vi "EG_G5210 Read Param.vi"(8 "error in (no error)":errorcluster, 9 "Énum":T3, 10 "LockInPar In":T1={"Sensitivity"=13, "Vernier Mode"=FALSE, "Vernier Value"=0, "Main Filter"=3, "Filter Freq (Hz)"=0.0, "Filter Mode"=1, " Line Notch"=3, "Reference"=1, "Reference Mode"=0, "Ref Phase (°)"=0.0, "Ref Freq (Hz)"=0.0, "Output Filter"=0, "Time Constant"=13, "Dynamic Res."=1, "X Offset"=FALSE, "X Offset Val %"=0.0, "Y Offset"=FALSE, "Y Offset Val %"=0.0, "Expand"=FALSE, "Osc Amp. (mV rms)"=0, "Int Osc (Hz)"=0.0, "Trigger Mode"=0, "Input Mode"=0, "Ovld Source"=0} caption="Lock-In Parameters In" {"Ovld Source" items=["None", "Y Channel", "X Channel", "PSD", "Input", "Ref Unlck"]; "Input Mode" items=["Current 10E8 A/V", "Current 10E6 A/V", "Voltage"]; "Trigger Mode" items=["Reference", "External", "Asynchronous", "Ratio", "8F"]; "Reference Mode" items=["F", "2F"]; "Reference" items=["External", "Internal"]; "Filter Mode" items=["Manual", "Automatic"]; "Line Notch" items=["Off", "120 Hz", "60 Hz", "Both"]; "Main Filter" items=["No Filter", "Notch", "Low Pass", "Band Pass"]; "Output Filter" items=["6dB", "12dB"]; "Time Constant" items=["1 ms", "3 ms", "10 ms", "30 ms", "100 ms", "300 ms", "1 s", "3 s", "10 s", "30 s", "100 s", "300 s", "1000 s", "3000 s"]; "Sensitivity" items=["100 nV", "300 nV", "1 µV", "3 µV", "10 µV", "30 µV", "100µV", "300 µV", "1 mV", "3 mV", "10 mV", "30 mV", "100 mV", "300 mV", "1 V", "3 V"]; "Dynamic Res." items=["Hi Stab", "Normal", "Hi Res"]}, 11 "Ressource VISA":refnum<visa-resource-name>="GPIB0::8::INSTR") -> (0 "error out":errorcluster, 1 "LockInPar":T1={"Sensitivity"=1, "Vernier Mode"=FALSE, "Vernier Value"=0, "Main Filter"=0, "Filter Freq (Hz)"=0.0, "Filter Mode"=0, " Line Notch"=0, "Reference"=0, "Reference Mode"=0, "Ref Phase (°)"=0.0, "Ref Freq (Hz)"=0.0, "Output Filter"=0, "Time Constant"=1, "Dynamic Res."=0, "X Offset"=FALSE, "X Offset Val %"=0.0, "Y Offset"=FALSE, "Y Offset Val %"=0.0, "Expand"=FALSE, "Osc Amp. (mV rms)"=0, "Int Osc (Hz)"=0.0, "Trigger Mode"=0, "Input Mode"=0, "Ovld Source"=0} caption="Lock-In Parameters Out" {"Ovld Source" items=["None", "Y Channel", "X Channel", "PSD", "Input", "Ref Unlck"]; "Input Mode" items=["Current 10E8 A/V", "Current 10E6 A/V", "Voltage"]; "Trigger Mode" items=["Reference", "External", "Asynchronous", "Ratio", "8F"]; "Reference Mode" items=["F", "2F"]; "Reference" items=["External", "Internal"]; "Filter Mode" items=["Manual", "Automatic"]; "Line Notch" items=["Off", "120 Hz", "60 Hz", "Both"]; "Main Filter" items=["No Filter", "Notch", "Low Pass", "Band Pass"]; "Output Filter" items=["6dB", "12dB"]; "Time Constant" items=["1 ms", "3 ms", "10 ms", "30 ms", "100 ms", "300 ms", "1 s", "3 s", "10 s", "30 s", "100 s", "300 s", "1000 s", "3000 s"]; "Sensitivity" items=["100 nV", "300 nV", "1 µV", "3 µV", "10 µV", "30 µV", "100µV", "300 µV", "1 mV", "3 mV", "10 mV", "30 mV", "100 mV", "300 mV", "1 V", "3 V"]; "Dynamic Res." items=["Hi Stab", "Normal", "Hi Res"]}, 2 "Params":string, 3 "Ressource VISA Out":refnum<visa-resource-name>="GPIB0::8::INSTR")   [LabVIEW 2019]
uses:
  <userlib>/EG_G 5210 LIA/LockInPar.ctl
  <userlib>/EG_G 5210 LIA/TrigMode.ctl
  <userlib>/EG_G 5210 LIA/ReadFunctions.ctl
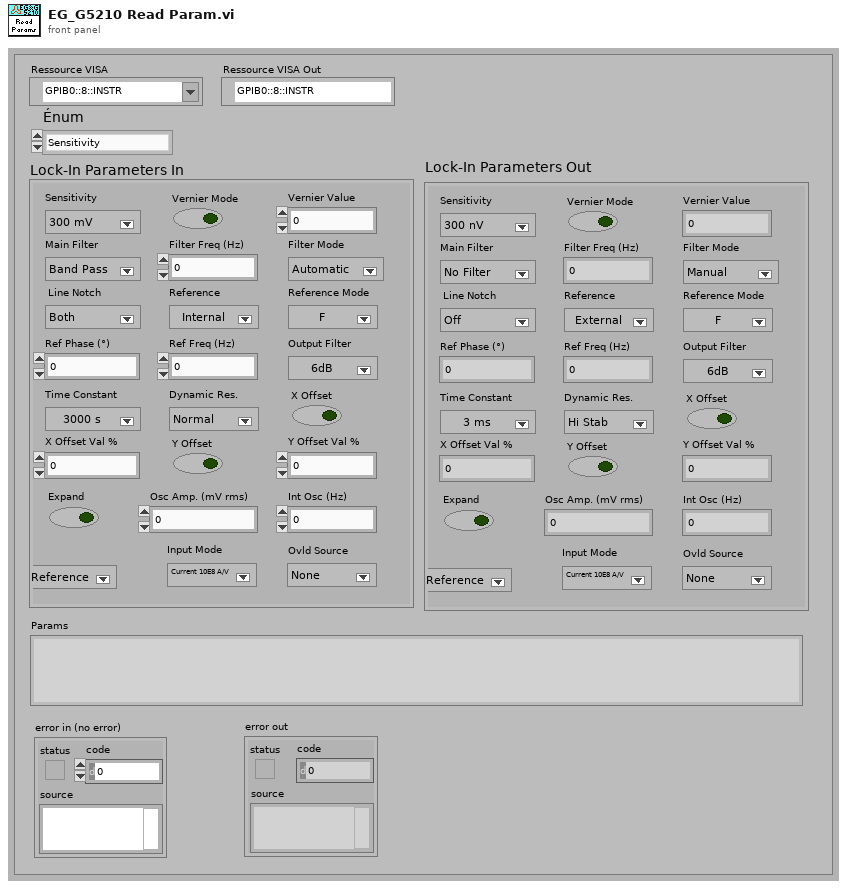
[diagram p1: front panel]
types:
  T1 = typedef "LockInPar.ctl" = cluster{"Sensitivity":u16, "Vernier Mode":bool, "Vernier Value":i32, "Main Filter":u16, "Filter Freq (Hz)":dbl, "Filter Mode":u16, " Line Notch":u16, "Reference":u16, "Reference Mode":u16, "Ref Phase (°)":dbl, "Ref Freq (Hz)":dbl, "Output Filter":u16, "Time Constant":u16, "Dynamic Res.":u16, "X Offset":bool, "X Offset Val %":dbl, "Y Offset":bool, "Y Offset Val %":dbl, "Expand":bool, "Osc Amp. (mV rms)":i32, "Int Osc (Hz)":dbl, "Trigger Mode":T2, "Input Mode":u16, "Ovld Source":u16}
  T2 = typedef "TrigMode.ctl" = u16
  T3 = typedef "ReadFunctions.ctl" = enum16{"Sensitivity", "Vernier Mode", "Main Filter", "Filter Mode", "Line Filter", "Ref Source", "Ref Mode", "Ref Phase", "Ref Frequency", "Output Filter", "Time Constant", "Dyn Reserve", "X Offset", "Y Offset", "Expand Mode", "Int Oscillator", "Oscillator Freq", "All params", "Overload Byte", "Trigger Mode", "Error"}
  T4 = enum16{"0.5 Hz to 12 Hz", "10 Hz to 120 Hz", "100 Hz to 1200 Hz", "1 kHz to 12 kHz", "10 kHz to 120 kHz"}
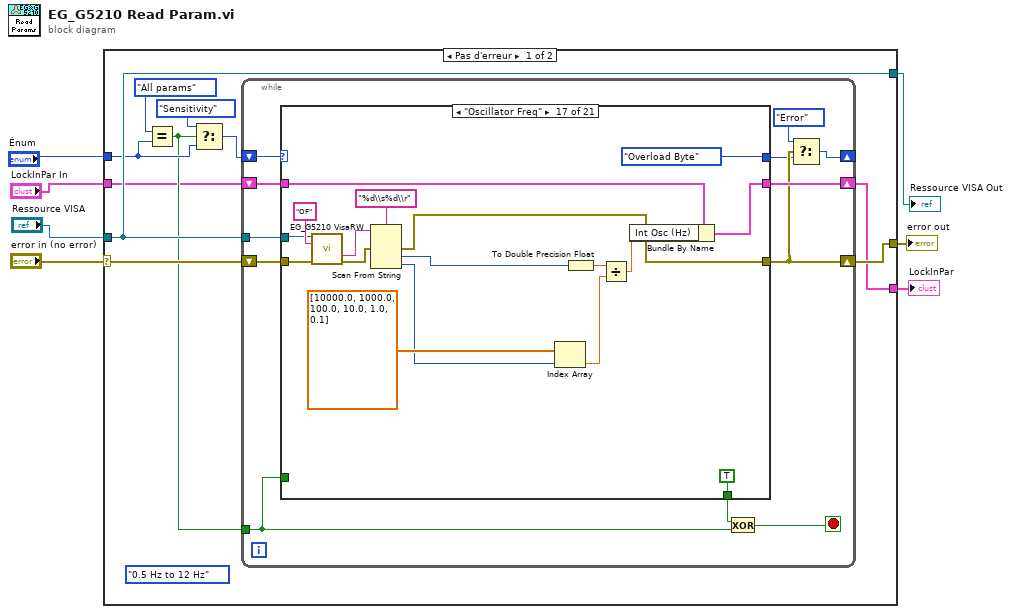
[diagram p0: block diagram]
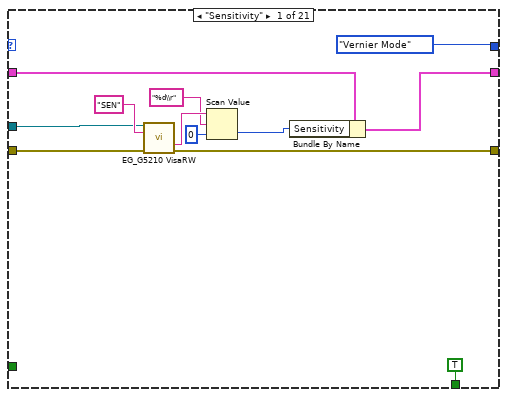
[diagram p2: hidden frame]
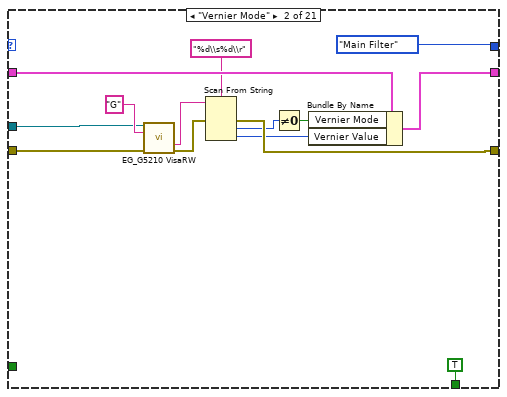
[diagram p3: hidden frame]
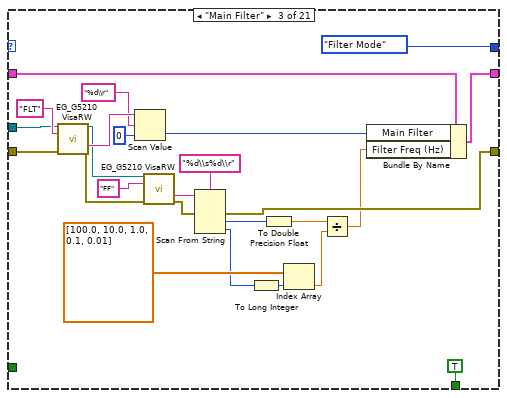
[diagram p4: hidden frame]
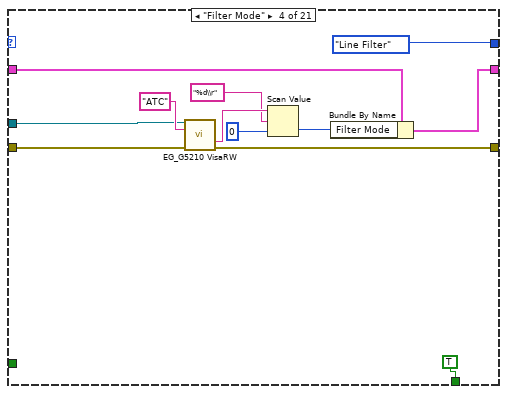
[diagram p5: hidden frame]
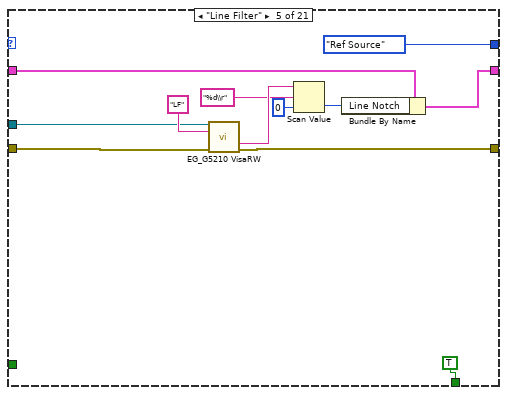
[diagram p6: hidden frame]
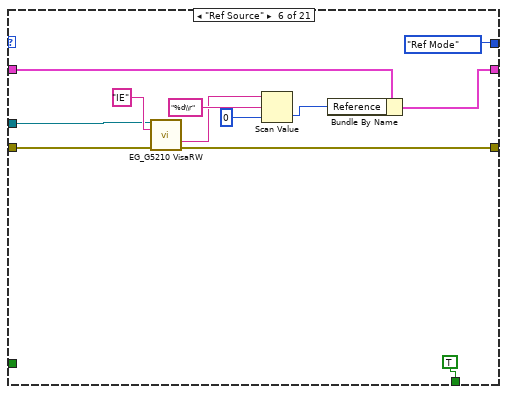
[diagram p7: hidden frame]
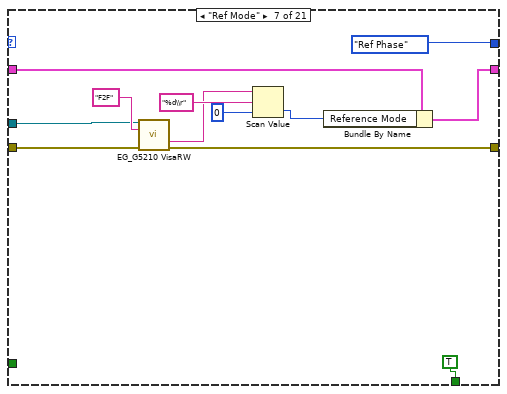
[diagram p8: hidden frame]
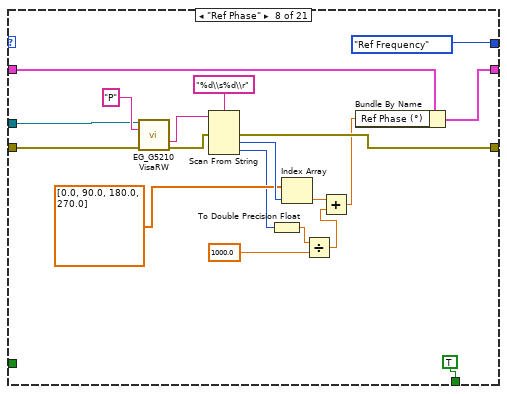
[diagram p9: hidden frame]
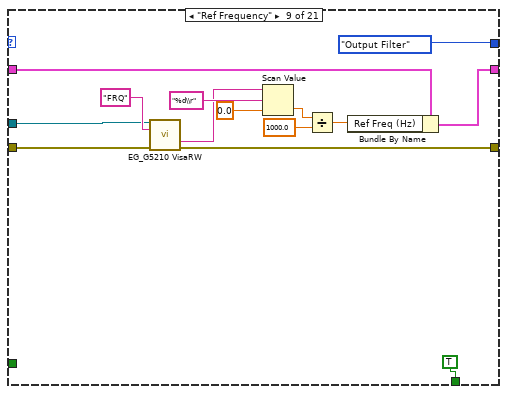
[diagram p10: hidden frame]
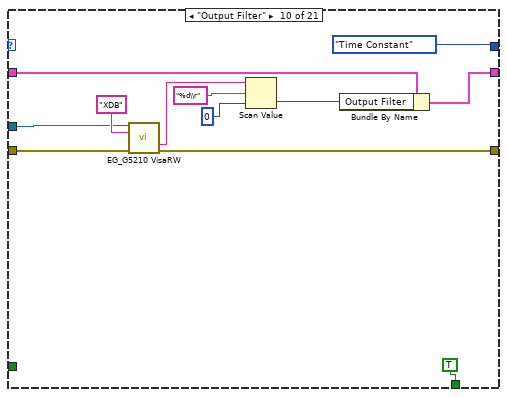
[diagram p11: hidden frame]
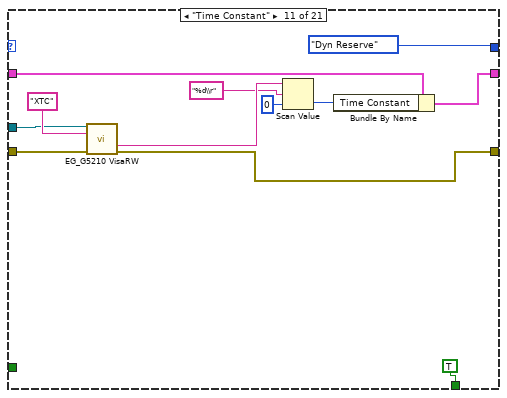
[diagram p12: hidden frame]
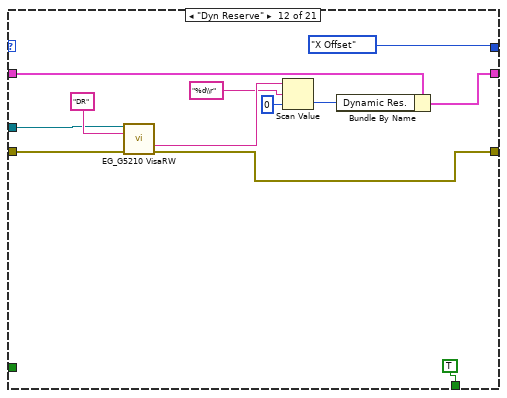
[diagram p13: hidden frame]
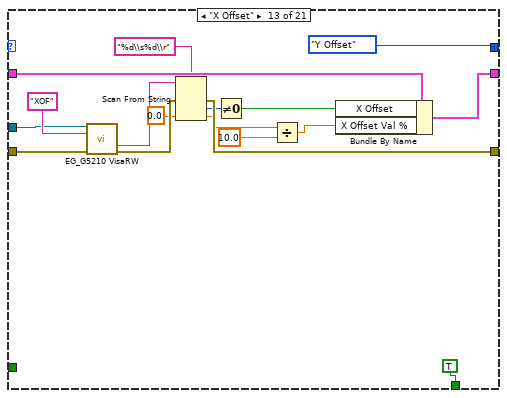
[diagram p14: hidden frame]
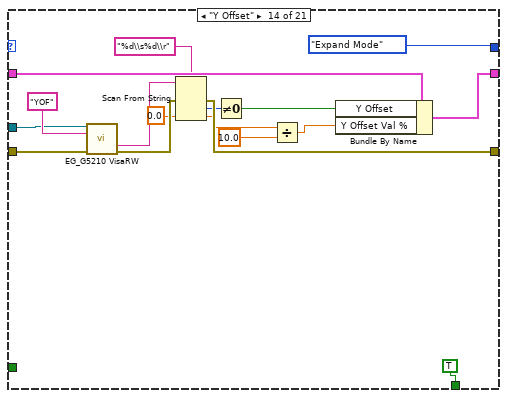
[diagram p15: hidden frame]
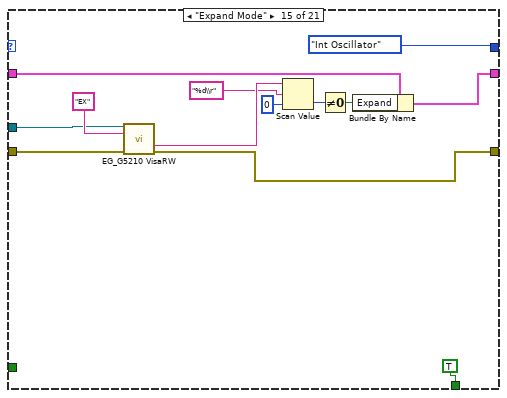
[diagram p16: hidden frame]
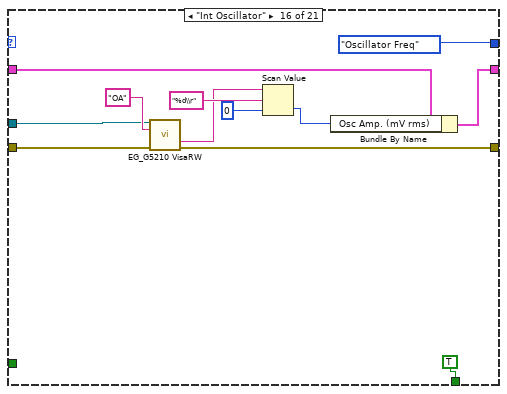
[diagram p17: hidden frame]
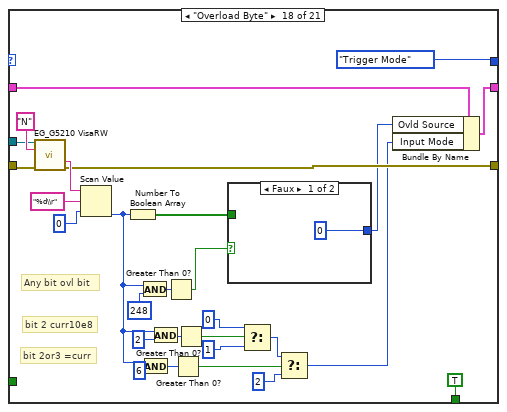
[diagram p18: hidden frame]
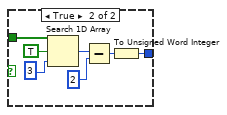
[diagram p19: hidden frame]
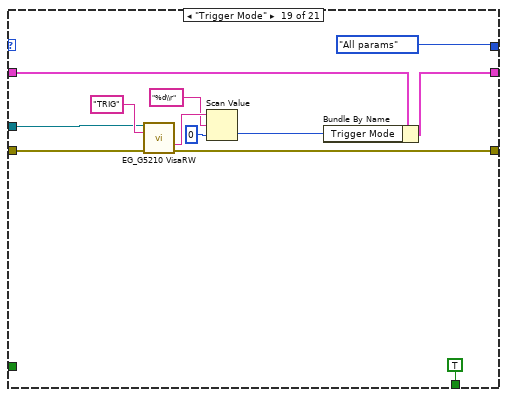
[diagram p20: hidden frame]
diagram:
  n1 = case shown="Pas d'erreur" "error in (no error)" {
    selector: "error in (no error)" -> [w16 w334]
    tunnel: [w17 w334] -> w6
    tunnel: [w15 w333] -> w5
    tunnel: "Ressource VISA" -> [w15 w333]
    tunnel: [w14 _] -> w3
    tunnel: "Énum" -> [w11 _]
    tunnel: "LockInPar In" -> [w8 _]
    frame No Error {
      (unwired) T4."0.5 Hz to 12 Hz"
      n2 = Equal?(x=ReadFunctions."All params" ("Énum"), y=w11) -> (x = y?=w9:bool)
      n3 = Select(t=ReadFunctions."Sensitivity" ("Énum"), s=w9, f=w11) -> (s? t:f=w10:T3)
      n4 = while {
        shift-right: [w19] -> _
        shift-left: w10 -> [w29]
        shift-right: [w21] -> w17
        shift-left: w16 -> [w28]
        tunnel: w15 -> [w27]
        shift-right: [w26] -> w14
        shift-left: w8 -> [w25]
        tunnel: w9 -> [w22]
        stop <- w23 stop-if-true
        n5 = case shown="\"Oscillator Freq\"" w29 {
          selector: w29 -> [_ _ _ _ _ _ _ _ _ _ _ _ _ _ _ _ _ _ _ _ w332]
          tunnel: w28 -> [w38 w54 w79 w91 w100 w115 w127 w146 w160 w172 w182 w194 w212 w229 w241 w255 w272 w298 w318 w326 w331]
          tunnel: [w36 w45 w59 w90 w94 w114 w126 w137 w159 w162 w174 w186 w205 w222 w233 w254 w258 w296 w316 w325 w331] -> w21
          tunnel: w27 -> [w37 w53 w78 w89 w101 w113 w125 w145 w158 w171 w181 w193 w211 w228 w240 w253 w271 w297 w317 _ _]
          tunnel: [ReadFunctions."Vernier Mode" ReadFunctions."Main Filter" ReadFunctions."Filter Mode" ReadFunctions."Line Filter" ReadFunctions."Ref Source" ReadFunctions."Ref Mode" ReadFunctions."Ref Phase" ReadFunctions."Ref Frequency" ReadFunctions."Output Filter" ReadFunctions."Time Constant" ReadFunctions."Dyn Reserve" ReadFunctions."X Offset" ReadFunctions."Y Offset" ReadFunctions."Expand Mode" ReadFunctions."Int Oscillator" ReadFunctions."Oscillator Freq" ReadFunctions."Overload Byte" ReadFunctions."Trigger Mode" ReadFunctions."All params" ReadFunctions."Vernier Mode" w332] -> w20
          tunnel: [TRUE TRUE TRUE TRUE TRUE TRUE TRUE TRUE TRUE TRUE TRUE TRUE TRUE TRUE TRUE TRUE TRUE TRUE TRUE FALSE w329] -> w24
          tunnel: w25 -> [w31 w49 w73 w83 w96 w110 w122 w142 w154 w166 w177 w189 w208 w225 w236 w249 w269 w292 w312 w322 w328]
          tunnel: [w32 w50 w57 w84 w97 w109 w121 w141 w155 w165 w176 w188 w207 w224 w235 w250 w268 w293 w313 w322 w328] -> w26
          tunnel: w22 -> [_ _ _ _ _ _ _ _ _ _ _ _ _ _ _ _ _ _ _ _ w330]
          frame "Sensitivity" {
            n6 = call <userlib>:"EG_G5210 VisaRW.vi"("VISA Rsrc"=w37, "ChaineCom"="SEN", "error in (no error)"=w38) -> ("ChaineRep"=w40:string, "error out"=w36:errorcluster)  [unwired: 9 in, 2 out]
            n7 = Scan Value(string=w40, format string="%d\\r" ("chaîne de format"), default (0 dbl)=u16 0 ("valeur par défaut (0 I32)")) -> (value=w33:u16)  [unwired: 1 out]
            n8 = Bundle By Name(cluster=w31, "Sensitivity"=w33) -> (w32:T1)
          }
          frame "Vernier Mode" {
            n9 = call <userlib>:"EG_G5210 VisaRW.vi"("VISA Rsrc"=w53, "ChaineCom"="G", "error in (no error)"=w54) -> ("ChaineRep"=w47:string, "error out"=w46:errorcluster)  [unwired: 9 in, 2 out]
            n10 = Scan From String(format string="%d\\s%d\\r" ("chaîne de format"), input string=w47, error in=w46) -> (error out=w45:errorcluster, output 1=w44:i32, output 2=w42:i32)  [unwired: 3 in, 2 out]
            n11 = Not Equal To 0?(x=w44) -> (x != 0?=w43:bool)
            n12 = Bundle By Name(cluster=w49, "Vernier Mode"=w43, "Vernier Value"=w42) -> (w50:T1)
          }
          frame "Main Filter" {
            n13 = call <userlib>:"EG_G5210 VisaRW.vi"("VISA Rsrc"=w78, "ChaineCom"="FLT", "error in (no error)"=w79) -> ("VISA Rsrc Out"=w71:refnum<visa-resource-name>, "ChaineRep"=w77:string, "error out"=w70:errorcluster)  [unwired: 9 in, 1 out]
            n14 = Scan Value(string=w77, format string="%d\\r" ("chaîne de format"), default (0 dbl)=u16 0 ("valeur par défaut (0 I32)")) -> (value=w72:u16)  [unwired: 1 out]
            n15 = call <userlib>:"EG_G5210 VisaRW.vi"("VISA Rsrc"=w71, "ChaineCom"="FF", "error in (no error)"=w70) -> ("ChaineRep"=w68:string, "error out"=w60:errorcluster)  [unwired: 9 in, 2 out]
            n16 = Scan From String(format string="%d\\s%d\\r" ("chaîne de format"), input string=w68, error in=w60) -> (error out=w59:errorcluster, output 1=w62:i32, output 2=w61:i32)  [unwired: 3 in, 2 out]
            n17 = To Long Integer(number=w61) -> (32bit integer=w65:i32)
            n18 = To Double Precision Float(number=w62) -> (double precision float=w63:dbl)
            n19 = Index Array(array=dbl[] [100.0, 10.0, 1.0, 0.1, 0.01], index=w65) -> (element=w66:dbl)
            n20 = Divide(x=w63, y=w66) -> (x/y=w56:dbl)
            n21 = Bundle By Name(cluster=w73, "Main Filter"=w72, "Filter Freq (Hz)"=w56) -> (w57:T1)
          }
          frame "Filter Mode" {
            n22 = call <userlib>:"EG_G5210 VisaRW.vi"("VISA Rsrc"=w89, "ChaineCom"="ATC", "error in (no error)"=w91) -> ("ChaineRep"=w88:string, "error out"=w90:errorcluster)  [unwired: 9 in, 2 out]
            n23 = Scan Value(string=w88, format string="%d\\r" ("chaîne de format"), default (0 dbl)=u16 0 ("valeur par défaut (0 I32)")) -> (value=w82:u16)  [unwired: 1 out]
            n24 = Bundle By Name(cluster=w83, "Filter Mode"=w82) -> (w84:T1)
          }
          frame "Line Filter" {
            n25 = call <userlib>:"EG_G5210 VisaRW.vi"("VISA Rsrc"=w101, "ChaineCom"="LF", "error in (no error)"=w100) -> ("ChaineRep"=w103:string, "error out"=w94:errorcluster)  [unwired: 9 in, 2 out]
            n26 = Scan Value(string=w103, format string="%d\\r" ("chaîne de format"), default (0 dbl)=u16 0 ("valeur par défaut (0 I32)")) -> (value=w95:u16)  [unwired: 1 out]
            n27 = Bundle By Name(cluster=w96, "Line Notch"=w95) -> (w97:T1)
          }
          frame "Ref Source" {
            n28 = call <userlib>:"EG_G5210 VisaRW.vi"("VISA Rsrc"=w113, "ChaineCom"="IE", "error in (no error)"=w115) -> ("ChaineRep"=w106:string, "error out"=w114:errorcluster)  [unwired: 9 in, 2 out]
            n29 = Scan Value(string=w106, format string="%d\\r" ("chaîne de format"), default (0 dbl)=u16 0 ("valeur par défaut (0 I32)")) -> (value=w105:u16)  [unwired: 1 out]
            n30 = Bundle By Name(cluster=w110, "Reference"=w105) -> (w109:T1)
          }
          frame "Ref Mode" {
            n31 = call <userlib>:"EG_G5210 VisaRW.vi"("VISA Rsrc"=w125, "ChaineCom"="F2F", "error in (no error)"=w127) -> ("ChaineRep"=w118:string, "error out"=w126:errorcluster)  [unwired: 9 in, 2 out]
            n32 = Scan Value(string=w118, format string="%d\\r" ("chaîne de format"), default (0 dbl)=u16 0 ("valeur par défaut (0 I32)")) -> (value=w117:u16)  [unwired: 1 out]
            n33 = Bundle By Name(cluster=w122, "Reference Mode"=w117) -> (w121:T1)
          }
          frame "Ref Phase" {
            n34 = call <userlib>:"EG_G5210 VisaRW.vi"("VISA Rsrc"=w145, "ChaineCom"="P", "error in (no error)"=w146) -> ("ChaineRep"=w139:string, "error out"=w138:errorcluster)  [unwired: 9 in, 2 out]
            n35 = Scan From String(format string="%d\\s%d\\r" ("chaîne de format"), input string=w139, error in=w138) -> (error out=w137:errorcluster, output 1=w136:i32, output 2=w131:i32)  [unwired: 3 in, 2 out]
            n36 = To Double Precision Float(number=w131) -> (double precision float=w132:dbl)
            n37 = Index Array(array=dbl[] [0.0, 90.0, 180.0, 270.0], index=w136) -> (element=w134:dbl)
            n38 = Divide(x=w132, y=1000.0) -> (x/y=w130:dbl)
            n39 = Add(x=w134, y=w130) -> (x+y=w129:dbl)
            n40 = Bundle By Name(cluster=w142, "Ref Phase (°)"=w129) -> (w141:T1)
          }
          frame "Ref Frequency" {
            n41 = call <userlib>:"EG_G5210 VisaRW.vi"("VISA Rsrc"=w158, "ChaineCom"="FRQ", "error in (no error)"=w160) -> ("ChaineRep"=w151:string, "error out"=w159:errorcluster)  [unwired: 9 in, 2 out]
            n42 = Scan Value(string=w151, format string="%d\\r" ("chaîne de format"), default (0 dbl)=0.0 ("valeur par défaut (0 I32)")) -> (value=w150:dbl)  [unwired: 1 out]
            n43 = Divide(x=w150, y=1000.0) -> (x/y=w149:dbl)
            n44 = Bundle By Name(cluster=w154, "Ref Freq (Hz)"=w149) -> (w155:T1)
          }
          frame "Output Filter" {
            n45 = call <userlib>:"EG_G5210 VisaRW.vi"("VISA Rsrc"=w171, "ChaineCom"="XDB", "error in (no error)"=w172) -> ("ChaineRep"=w170:string, "error out"=w162:errorcluster)  [unwired: 9 in, 2 out]
            n46 = Scan Value(string=w170, format string="%d\\r" ("chaîne de format"), default (0 dbl)=u16 0 ("valeur par défaut (0 I32)")) -> (value=w164:u16)  [unwired: 1 out]
            n47 = Bundle By Name(cluster=w166, "Output Filter"=w164) -> (w165:T1)
          }
          frame "Time Constant" {
            n48 = call <userlib>:"EG_G5210 VisaRW.vi"("VISA Rsrc"=w181, "ChaineCom"="XTC", "error in (no error)"=w182) -> ("ChaineRep"=w184:string, "error out"=w174:errorcluster)  [unwired: 9 in, 2 out]
            n49 = Scan Value(string=w184, format string="%d\\r" ("chaîne de format"), default (0 dbl)=u16 0 ("valeur par défaut (0 I32)")) -> (value=w178:u16)  [unwired: 1 out]
            n50 = Bundle By Name(cluster=w177, "Time Constant"=w178) -> (w176:T1)
          }
          frame "Dyn Reserve" {
            n51 = call <userlib>:"EG_G5210 VisaRW.vi"("VISA Rsrc"=w193, "ChaineCom"="DR", "error in (no error)"=w194) -> ("ChaineRep"=w196:string, "error out"=w186:errorcluster)  [unwired: 9 in, 2 out]
            n52 = Scan Value(string=w196, format string="%d\\r" ("chaîne de format"), default (0 dbl)=u16 0 ("valeur par défaut (0 I32)")) -> (value=w190:u16)  [unwired: 1 out]
            n53 = Bundle By Name(cluster=w189, "Dynamic Res."=w190) -> (w188:T1)
          }
          frame "X Offset" {
            n54 = call <userlib>:"EG_G5210 VisaRW.vi"("VISA Rsrc"=w211, "ChaineCom"="XOF", "error in (no error)"=w212) -> ("ChaineRep"=w213:string, "error out"=w206:errorcluster)  [unwired: 9 in, 2 out]
            n55 = Scan From String(format string="%d\\s%d\\r" ("chaîne de format"), input string=w213, error in=w206, default 2=0.0 ("valeur par défaut (0 I32)")) -> (error out=w205:errorcluster, output 1=w204:i32, output 2=w200:dbl)  [unwired: 2 in, 2 out]
            n56 = Not Equal To 0?(x=w204) -> (x != 0?=w202:bool)
            n57 = Divide(x=w200, y=10.0) -> (x/y=w198:dbl)
            n58 = Bundle By Name(cluster=w208, "X Offset"=w202, "X Offset Val %"=w198) -> (w207:T1)
          }
          frame "Y Offset" {
            n59 = call <userlib>:"EG_G5210 VisaRW.vi"("VISA Rsrc"=w228, "ChaineCom"="YOF", "error in (no error)"=w229) -> ("ChaineRep"=w230:string, "error out"=w223:errorcluster)  [unwired: 9 in, 2 out]
            n60 = Scan From String(format string="%d\\s%d\\r" ("chaîne de format"), input string=w230, error in=w223, default 2=0.0 ("valeur par défaut (0 I32)")) -> (error out=w222:errorcluster, output 1=w221:i32, output 2=w217:dbl)  [unwired: 2 in, 2 out]
            n61 = Not Equal To 0?(x=w221) -> (x != 0?=w219:bool)
            n62 = Divide(x=w217, y=10.0) -> (x/y=w215:dbl)
            n63 = Bundle By Name(cluster=w225, "Y Offset"=w219, "Y Offset Val %"=w215) -> (w224:T1)
          }
          frame "Expand Mode" {
            n64 = call <userlib>:"EG_G5210 VisaRW.vi"("VISA Rsrc"=w240, "ChaineCom"="EX", "error in (no error)"=w241) -> ("ChaineRep"=w243:string, "error out"=w233:errorcluster)  [unwired: 9 in, 2 out]
            n65 = Scan Value(string=w243, format string="%d\\r" ("chaîne de format"), default (0 dbl)=u16 0 ("valeur par défaut (0 I32)")) -> (value=w237:u16)  [unwired: 1 out]
            n66 = Not Equal To 0?(x=w237) -> (x != 0?=w232:bool)
            n67 = Bundle By Name(cluster=w236, "Expand"=w232) -> (w235:T1)
          }
          frame "Int Oscillator" {
            n68 = call <userlib>:"EG_G5210 VisaRW.vi"("VISA Rsrc"=w253, "ChaineCom"="OA", "error in (no error)"=w255) -> ("ChaineRep"=w246:string, "error out"=w254:errorcluster)  [unwired: 9 in, 2 out]
            n69 = Scan Value(string=w246, format string="%d\\r" ("chaîne de format"), default (0 dbl)=0 ("valeur par défaut (0 I32)")) -> (value=w245:i32)  [unwired: 1 out]
            n70 = Bundle By Name(cluster=w249, "Osc Amp. (mV rms)"=w245) -> (w250:T1)
          }
          frame "Oscillator Freq" {
            n71 = call <userlib>:"EG_G5210 VisaRW.vi"("VISA Rsrc"=w271, "ChaineCom"="OF", "error in (no error)"=w272) -> ("ChaineRep"=w266:string, "error out"=w265:errorcluster)  [unwired: 9 in, 2 out]
            n72 = Scan From String(format string="%d\\s%d\\r" ("chaîne de format"), input string=w266, error in=w265) -> (error out=w258:errorcluster, output 1=w257:i32, output 2=w259:i32)  [unwired: 3 in, 2 out]
            n73 = Index Array(array=dbl[] [10000.0, 1000.0, 100.0, 10.0, 1.0, 0.1], index=w259) -> (element=w262:dbl)
            n74 = To Double Precision Float(number=w257) -> (double precision float=w264:dbl)
            n75 = Divide(x=w264, y=w262) -> (x/y=w261:dbl)
            n76 = Bundle By Name(cluster=w269, "Int Osc (Hz)"=w261) -> (w268:T1)
          }
          frame "Overload Byte" {
            # "Any bit ovl bit"
            # "bit 2or3 =curr"
            # "bit 2 curr10e8"
            n77 = call <userlib>:"EG_G5210 VisaRW.vi"("VISA Rsrc"=w297, "ChaineCom"="N", "error in (no error)"=w298) -> ("ChaineRep"=w300:string, "error out"=w296:errorcluster)  [unwired: 9 in, 2 out]
            n78 = Scan Value(string=w300, format string="%d\\r" ("chaîne de format"), default (0 dbl)=u16 0 ("valeur par défaut (0 I32)")) -> (value=w277:u16)  [unwired: 1 out]
            n79 = Number To Boolean Array(number=w277) -> (Boolean array=w276:bool[])
            n80 = And(x=w277, y=u16 248) -> (x .and. y?=w279:u16)
            n81 = And(x=w277, y=u16 6) -> (x .and. y?=w287:u16)
            n82 = And(x=w277, y=u16 2) -> (x .and. y?=w286:u16)
            n83 = Greater Than 0?(x=w279) -> (x > 0?=w275:bool)
            n84 = Greater Than 0?(x=w287) -> (x > 0?=w289:bool)
            n85 = Greater Than 0?(x=w286) -> (x > 0?=w284:bool)
            n86 = case shown="Faux" w275 {
              tunnel: w276 -> [_ w308]
              tunnel: [u16 0 w306] -> w274
              frame False {
              }
              frame True {
                n87 = Search 1D Array(1D array=w308, element=TRUE ("élément"), start index (0)=3 ("indice de départ (0)")) -> (index of element=w305:i32)
                n88 = Subtract(x=w305, y=2) -> (x-y=w304:i32)
                n89 = To Unsigned Word Integer(number=w304) -> (unsigned 16bit integer=w306:u16)
              }
            }
            n90 = Select(t=u16 0 ("Input Mode"), s=w284, f=u16 1 ("Input Mode")) -> (s? t:f=w281:u16)
            n91 = Select(t=w281, s=w289, f=u16 2 ("Input Mode")) -> (s? t:f=w280:u16)
            n92 = Bundle By Name(cluster=w292, "Ovld Source"=w274, "Input Mode"=w280) -> (w293:T1)
          }
          frame "Trigger Mode" {
            n93 = call <userlib>:"EG_G5210 VisaRW.vi"("VISA Rsrc"=w317, "ChaineCom"="TRIG", "error in (no error)"=w318) -> ("ChaineRep"=w320:string, "error out"=w316:errorcluster)  [unwired: 9 in, 2 out]
            n94 = Scan Value(string=w320, format string="%d\\r" ("chaîne de format"), default (0 dbl)=u16 0 ("valeur par défaut (0 I32)")) -> (value=w310:u16)  [unwired: 1 out]
            n95 = Bundle By Name(cluster=w312, "Trigger Mode"=w310) -> (w313:T1)
          }
          frame "All params" {
            n96 = call <userlib>:"EG_G5210 ParString.vi"("entrée d'erreur (pas d'erreur)"=w326, "LockInPar"=w322) -> ("sortie d'erreur"=w325:errorcluster, "Chaîne"=→"Params":string)  [unwired: 8 in]
          }
          frame "Error", Default {
            n97 = Not(x=w330) -> (.not. x?=w329:bool)
          }
        }
        n98 = Exclusive Or(1:w22, 2:w24) -> (0:w23:bool)
        n99 = Select(t=ReadFunctions."Error", s=w21, f=w20) -> (s? t:f=w19:T3)
      }
    }
    frame Error {
    }
  }
  "error out" <- w6
  "Ressource VISA Out" <- w5
  "LockInPar" <- w3
